vi "CRYUpdate Calibration Date.vi"(11 "Calibration In":T1 {"Calibration 2D"."Sens Curve"."Z data" items=["dB", "Lin"]; "Calibration 2D"."Sens Curve"."X data" items=["dB", "Lin"]; "Calibration 2D"."Sens Curve"."Y data" items=["dB", "Lin"]; "Calibration 2D"."Sens Curve"."Z dB ref" format="%.1f"; "Calibration 2D"."Sens Curve"."Z axis" items=["Log", "Lin"]; "Calibration 2D"."Sens Curve"."X dB ref" format="%.1f"; "Calibration 2D"."Sens Curve"."X axis" items=["Log", "Lin"]; "Calibration 2D"."Sens Curve"."Y axis" items=["Log", "Lin"]; "Calibration 2D"."Sens Curve"."Y dB ref" format="%.1f"; "Calibration 2D"."Sens Curve"."Curve"."z" format="%.2f"; "Calibration 2D"."Sens Curve"."Curve"."y" format="%.2f"; "Calibration 2D"."Sens Curve"."Curve"."x" format="%.2f"; "Calibration 2D"."EQ Curve"."Z data" items=["dB", "Lin"]; "Calibration 2D"."EQ Curve"."X data" items=["dB", "Lin"]; "Calibration 2D"."EQ Curve"."Y data" items=["dB", "Lin"]; "Calibration 2D"."EQ Curve"."Z dB ref" format="%.1f"; "Calibration 2D"."EQ Curve"."Z axis" items=["Log", "Lin"]; "Calibration 2D"."EQ Curve"."X dB ref" format="%.1f"; "Calibration 2D"."EQ Curve"."X axis" items=["Log", "Lin"]; "Calibration 2D"."EQ Curve"."Y axis" items=["Log", "Lin"]; "Calibration 2D"."EQ Curve"."Y dB ref" format="%.1f"; "Calibration 2D"."EQ Curve"."Curve"."z" format="%.2f"; "Calibration 2D"."EQ Curve"."Curve"."y" format="%.2f"; "Calibration 2D"."EQ Curve"."Curve"."x" format="%.2f"; "Calibration 2D"."Corr Curve"."Z data" items=["dB", "Lin"]; "Calibration 2D"."Corr Curve"."X data" items=["dB", "Lin"]; "Calibration 2D"."Corr Curve"."Y data" items=["dB", "Lin"]; "Calibration 2D"."Corr Curve"."Z dB ref" format="%.1f"; "Calibration 2D"."Corr Curve"."Z axis" items=["Log", "Lin"]; "Calibration 2D"."Corr Curve"."X dB ref" format="%.1f"; "Calibration 2D"."Corr Curve"."X axis" items=["Log", "Lin"]; "Calibration 2D"."Corr Curve"."Y axis" items=["Log", "Lin"]; "Calibration 2D"."Corr Curve"."Y dB ref" format="%.1f"; "Calibration 2D"."Corr Curve"."Curve"."z" format="%.2f"; "Calibration 2D"."Corr Curve"."Curve"."y" format="%.2f"; "Calibration 2D"."Corr Curve"."Curve"."x" format="%.2f"; "Calibration 2D"."Calibration"."EQ Step size" items=["R10", "R20", "R40", "R80", "User"]; "Calibration 2D"."Calibration"."Corr Step size" items=["R10", "R20", "R40", "R80", "User"]}) -> (3 "Calibration Out":T1 {"Calibration 2D"."Sens Curve"."Z data" items=["dB", "Lin"]; "Calibration 2D"."Sens Curve"."X data" items=["dB", "Lin"]; "Calibration 2D"."Sens Curve"."Y data" items=["dB", "Lin"]; "Calibration 2D"."Sens Curve"."Z dB ref" format="%.1f"; "Calibration 2D"."Sens Curve"."Z axis" items=["Log", "Lin"]; "Calibration 2D"."Sens Curve"."X dB ref" format="%.1f"; "Calibration 2D"."Sens Curve"."X axis" items=["Log", "Lin"]; "Calibration 2D"."Sens Curve"."Y axis" items=["Log", "Lin"]; "Calibration 2D"."Sens Curve"."Y dB ref" format="%.1f"; "Calibration 2D"."Sens Curve"."Curve"."z" format="%.2f"; "Calibration 2D"."Sens Curve"."Curve"."y" format="%.2f"; "Calibration 2D"."Sens Curve"."Curve"."x" format="%.2f"; "Calibration 2D"."EQ Curve"."Z data" items=["dB", "Lin"]; "Calibration 2D"."EQ Curve"."X data" items=["dB", "Lin"]; "Calibration 2D"."EQ Curve"."Y data" items=["dB", "Lin"]; "Calibration 2D"."EQ Curve"."Z dB ref" format="%.1f"; "Calibration 2D"."EQ Curve"."Z axis" items=["Log", "Lin"]; "Calibration 2D"."EQ Curve"."X dB ref" format="%.1f"; "Calibration 2D"."EQ Curve"."X axis" items=["Log", "Lin"]; "Calibration 2D"."EQ Curve"."Y axis" items=["Log", "Lin"]; "Calibration 2D"."EQ Curve"."Y dB ref" format="%.1f"; "Calibration 2D"."EQ Curve"."Curve"."z" format="%.2f"; "Calibration 2D"."EQ Curve"."Curve"."y" format="%.2f"; "Calibration 2D"."EQ Curve"."Curve"."x" format="%.2f"; "Calibration 2D"."Corr Curve"."Z data" items=["dB", "Lin"]; "Calibration 2D"."Corr Curve"."X data" items=["dB", "Lin"]; "Calibration 2D"."Corr Curve"."Y data" items=["dB", "Lin"]; "Calibration 2D"."Corr Curve"."Z dB ref" format="%.1f"; "Calibration 2D"."Corr Curve"."Z axis" items=["Log", "Lin"]; "Calibration 2D"."Corr Curve"."X dB ref" format="%.1f"; "Calibration 2D"."Corr Curve"."X axis" items=["Log", "Lin"]; "Calibration 2D"."Corr Curve"."Y axis" items=["Log", "Lin"]; "Calibration 2D"."Corr Curve"."Y dB ref" format="%.1f"; "Calibration 2D"."Corr Curve"."Curve"."z" format="%.2f"; "Calibration 2D"."Corr Curve"."Curve"."y" format="%.2f"; "Calibration 2D"."Corr Curve"."Curve"."x" format="%.2f"; "Calibration 2D"."Calibration"."EQ Step size" items=["R10", "R20", "R40", "R80", "User"]; "Calibration 2D"."Calibration"."Corr Step size" items=["R10", "R20", "R40", "R80", "User"]})   [LabVIEW 2013]
uses:
  Typedef Control/CRYCalibration All Cluster.ctl
  Typedef Control/CRYCalibration 2DCluster.ctl
  Typedef Control/CRYCalibration Cluster.ctl
  Typedef Control/CRYData Cluster.ctl
  CRYProject/CRYProject Editor Global.vi
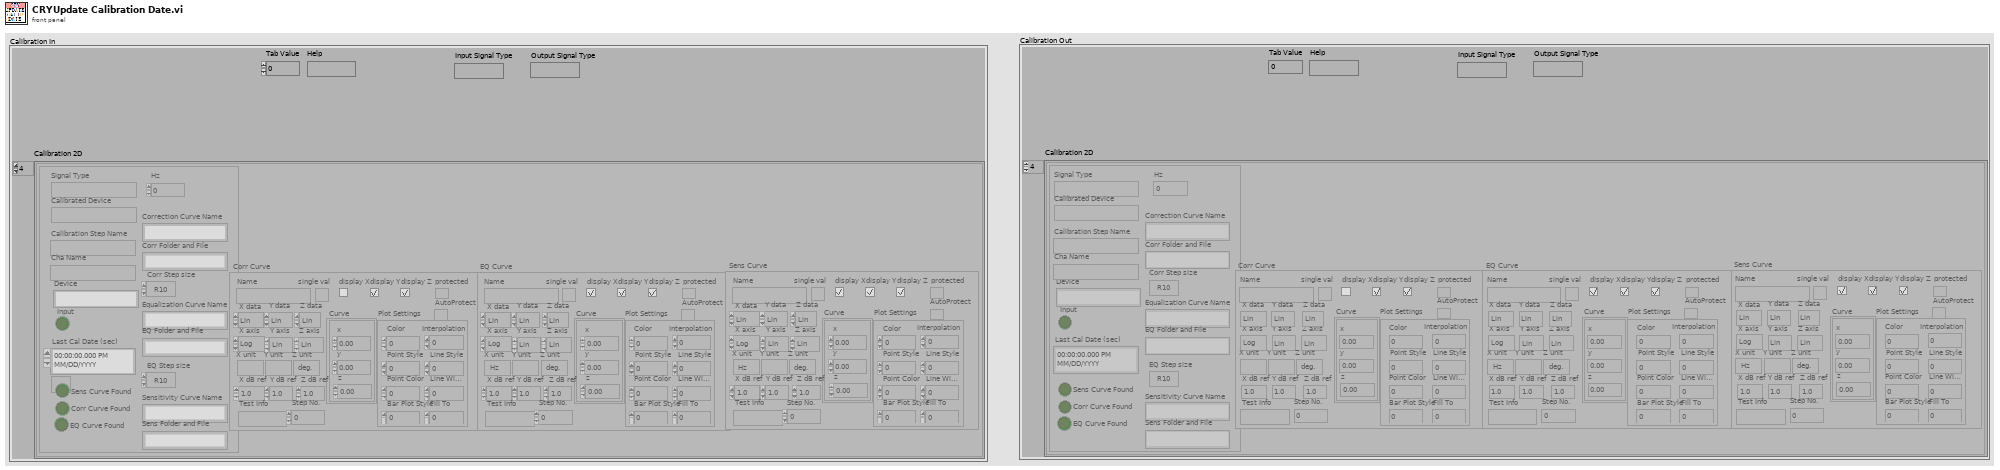
[diagram p1: front panel]
types:
  T1 = typedef "CRYCalibration All Cluster.ctl" = cluster{"Calibration 2D":T2[], "Help":string, "Tab Value":i32, "Input Signal Type":string, "Output Signal Type":string}
  T2 = typedef "CRYCalibration 2DCluster.ctl" = cluster{"Calibration":T3, "Corr Curve":T4, "EQ Curve":T4, "Sens Curve":T4}
  T3 = typedef "CRYCalibration Cluster.ctl" = cluster{"Calibration Step Name":string, "Device":string, "Correction Curve Name":string, "Equalization Curve Name":string, "Sensitivity Curve Name":string, "Corr Folder and File":string, "EQ Folder and File":string, "Sens Folder and File":string, "Corr Step size":u16, "EQ Step size":u16, "Input":bool, "Last Cal Date (sec)":timestamp, "Cha Name":string, "Corr Curve Found":bool, "EQ Curve Found":bool, "Sens Curve Found":bool, "Signal Type":string, "Calibrated Device":string, "Hz":u32}
  T4 = typedef "CRYData Cluster.ctl" = cluster{"Name":string, "Curve":cluster{"x":dbl, "y":dbl, "z":dbl}[], "X data":u16, "Y data":u16, "Z data":u16, "X axis":u16, "Y axis":u16, "Z axis":u16, "X unit":string, "Y unit":string, "Z unit":string, "X dB ref":dbl, "Y dB ref":dbl, "Z dB ref":dbl, "single val":bool, "protected":bool, "display X":bool, "display Y":bool, "display Z":bool, "Test Info":string, "Step No.":i32, "Plot Settings":cluster{"Color":u32, "Interpolation":u8, "Point Style":u8, "Line Style":u8, "Point Color":u32, "Line Width":u8, "Bar Plot Style":u8, "Fill To":i16}, "AutoProtect":bool}
  T5 = typedef "CRYStep.ctl" = cluster{"No.VI":i32, "Category":string, "StepName":string, "Seq setup flattened":string, "Comment":string, "Steps config.":bool[], "Jump config":i32[], "Start":dbl, "Increment":dbl, "Name":string, "Unit":string, "Y data":u16, "Y prefix":string, "Y dB ref":dbl, "Y unit":string, "Repeat State Array":cluster{"Start":dbl, "Increment":dbl, "Count":i32, "Num":i32}[]}
  T6 = cluster{"Calibration":cluster{"Calibration Step Name":bool, "Device":bool, "Correction Curve Name":bool, "Equalization Curve Name":bool, "Sensitivity Curve Name":bool, "Corr Folder and File":bool, "EQ Folder and File":bool, "Sens Folder and File":bool, "Corr Step size":bool, "EQ Step size":bool, "Input":bool, "Last Cal Date (sec)":bool, "Cha Name":bool, "Corr Curve Found":bool, "EQ Curve Found":bool, "Sens Curve Found":bool, "Signal Type":bool, "Calibrated Device":bool, "Hz":bool}, "Corr Curve":cluster{"Name":bool, "Curve":cluster{"x":bool, "y":bool, "z":bool}[], "X data":bool, "Y data":bool, "Z data":bool, "X axis":bool, "Y axis":bool, "Z axis":bool, "X unit":bool, "Y unit":bool, "Z unit":bool, "X dB ref":bool, "Y dB ref":bool, "Z dB ref":bool, "single val":bool, "protected":bool, "display X":bool, "display Y":bool, "display Z":bool, "Test Info":bool, "Step No.":bool, "Plot Settings":cluster{"Color":bool, "Interpolation":bool, "Point Style":bool, "Line Style":bool, "Point Color":bool, "Line Width":bool, "Bar Plot Style":bool, "Fill To":bool}, "AutoProtect":bool}, "EQ Curve":cluster{"Name":bool, "Curve":cluster{"x":bool, "y":bool, "z":bool}[], "X data":bool, "Y data":bool, "Z data":bool, "X axis":bool, "Y axis":bool, "Z axis":bool, "X unit":bool, "Y unit":bool, "Z unit":bool, "X dB ref":bool, "Y dB ref":bool, "Z dB ref":bool, "single val":bool, "protected":bool, "display X":bool, "display Y":bool, "display Z":bool, "Test Info":bool, "Step No.":bool, "Plot Settings":cluster{"Color":bool, "Interpolation":bool, "Point Style":bool, "Line Style":bool, "Point Color":bool, "Line Width":bool, "Bar Plot Style":bool, "Fill To":bool}, "AutoProtect":bool}, "Sens Curve":cluster{"Name":bool, "Curve":cluster{"x":bool, "y":bool, "z":bool}[], "X data":bool, "Y data":bool, "Z data":bool, "X axis":bool, "Y axis":bool, "Z axis":bool, "X unit":bool, "Y unit":bool, "Z unit":bool, "X dB ref":bool, "Y dB ref":bool, "Z dB ref":bool, "single val":bool, "protected":bool, "display X":bool, "display Y":bool, "display Z":bool, "Test Info":bool, "Step No.":bool, "Plot Settings":cluster{"Color":bool, "Interpolation":bool, "Point Style":bool, "Line Style":bool, "Point Color":bool, "Line Width":bool, "Bar Plot Style":bool, "Fill To":bool}, "AutoProtect":bool}}
  T7 = cluster{"Calibration Step Name":bool, "Device":bool, "Correction Curve Name":bool, "Equalization Curve Name":bool, "Sensitivity Curve Name":bool, "Corr Folder and File":bool, "EQ Folder and File":bool, "Sens Folder and File":bool, "Corr Step size":bool, "EQ Step size":bool, "Input":bool, "Last Cal Date (sec)":bool, "Cha Name":bool, "Corr Curve Found":bool, "EQ Curve Found":bool, "Sens Curve Found":bool, "Signal Type":bool, "Calibrated Device":bool, "Hz":bool}
  T8 = cluster{"Name":bool, "Curve":cluster{"x":bool, "y":bool, "z":bool}[], "X data":bool, "Y data":bool, "Z data":bool, "X axis":bool, "Y axis":bool, "Z axis":bool, "X unit":bool, "Y unit":bool, "Z unit":bool, "X dB ref":bool, "Y dB ref":bool, "Z dB ref":bool, "single val":bool, "protected":bool, "display X":bool, "display Y":bool, "display Z":bool, "Test Info":bool, "Step No.":bool, "Plot Settings":cluster{"Color":bool, "Interpolation":bool, "Point Style":bool, "Line Style":bool, "Point Color":bool, "Line Width":bool, "Bar Plot Style":bool, "Fill To":bool}, "AutoProtect":bool}
  T9 = cluster{"Color":bool, "Interpolation":bool, "Point Style":bool, "Line Style":bool, "Point Color":bool, "Line Width":bool, "Bar Plot Style":bool, "Fill To":bool}
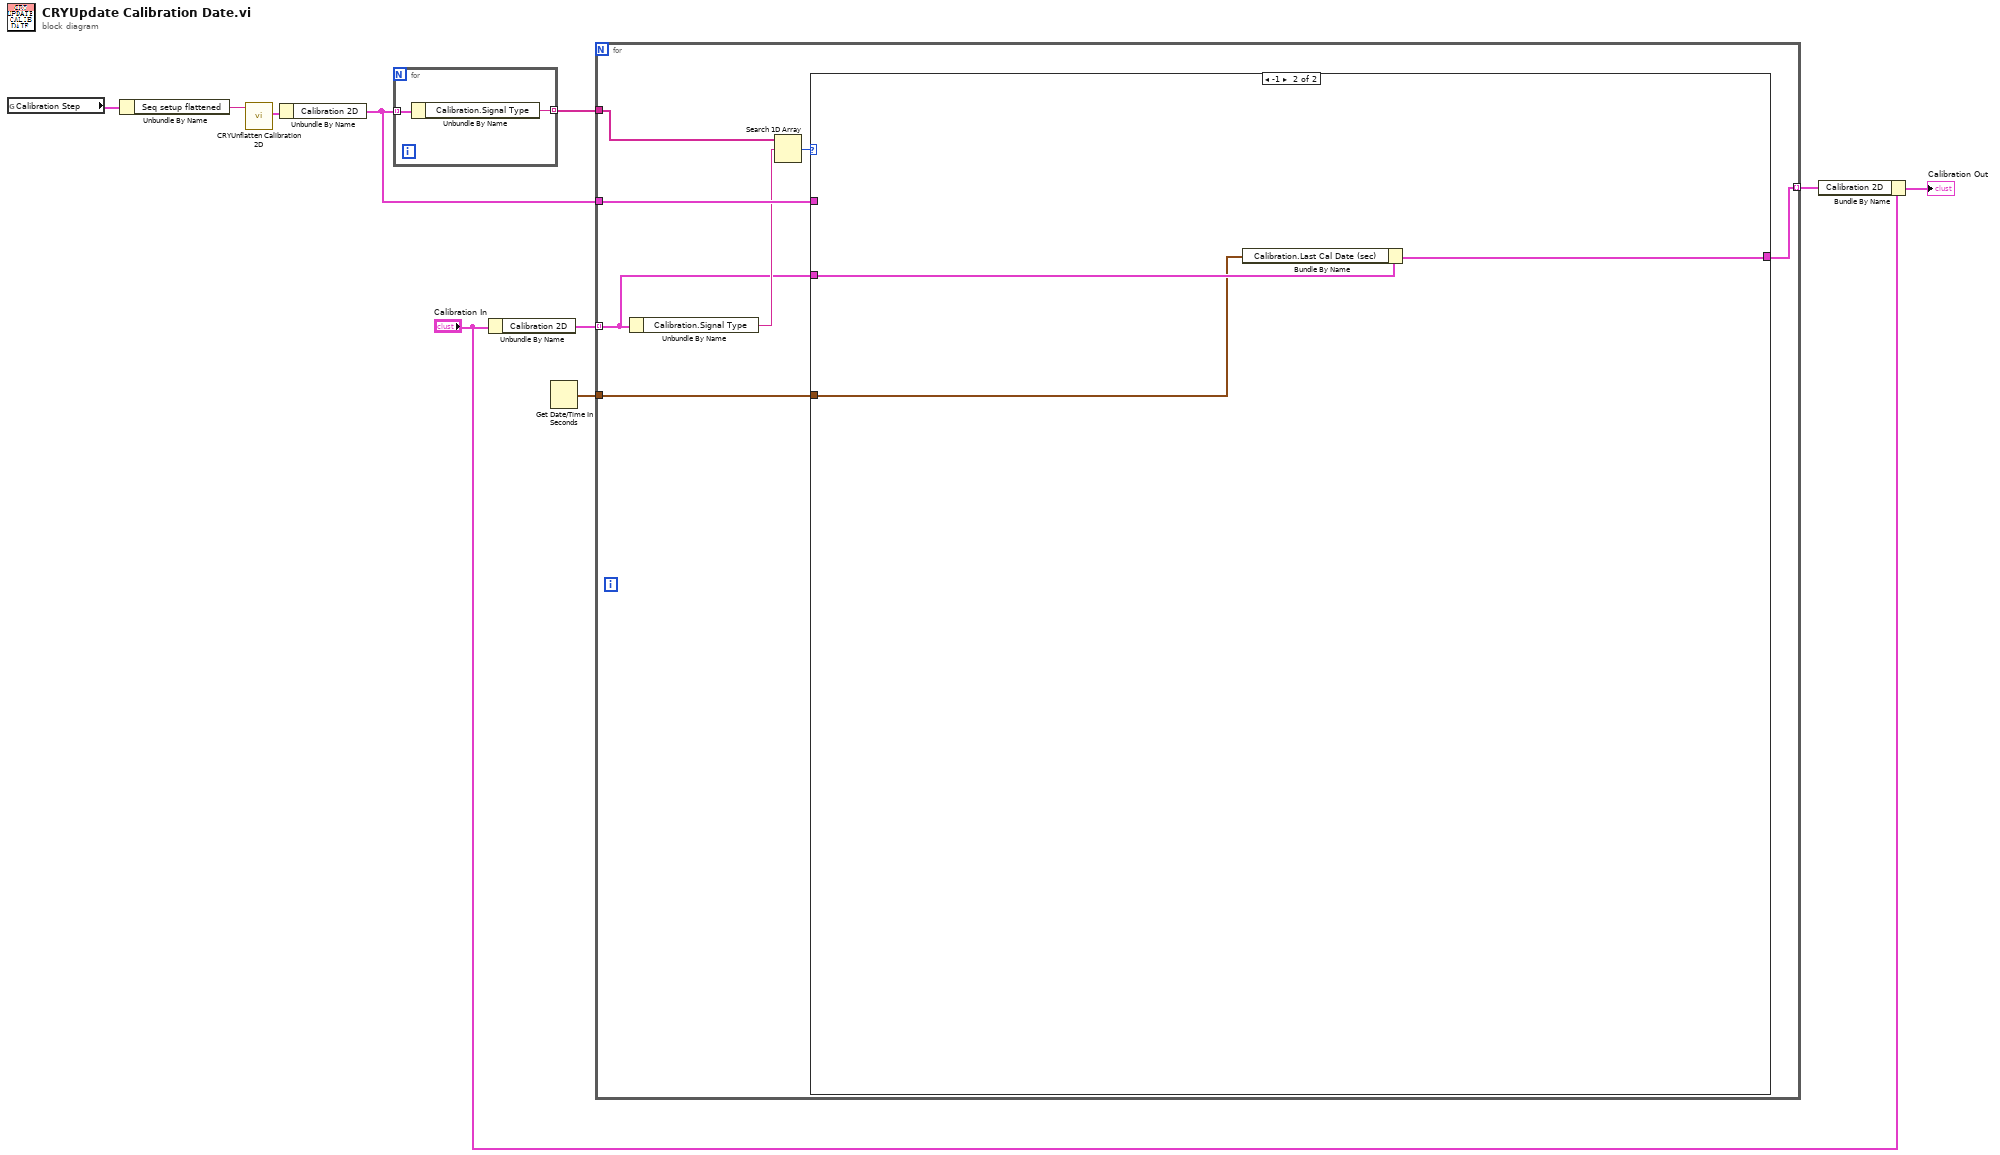
[diagram p0: block diagram]
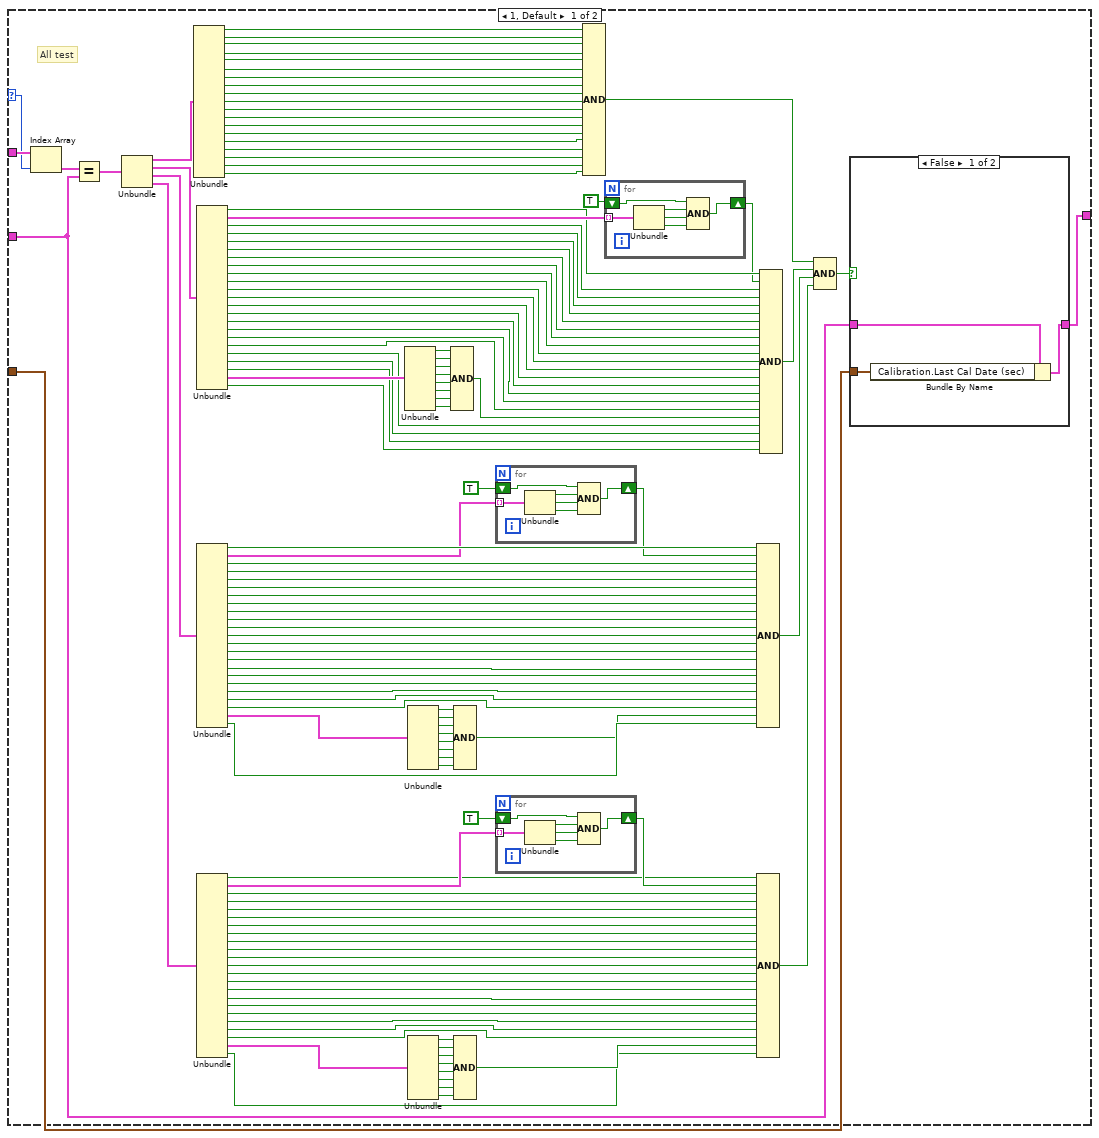
[diagram p2: hidden frame]
diagram:
  n1 = global read "CRYProject Editor Global.vi" "Calibration Step"() -> (w10:T5)
  n2 = Unbundle By Name(w10) -> ("Seq setup flattened"=w9:string)
  n3 = call "CRYUnflatten Calibration 2D.vi"("Flattened Calibration"=w9) -> ("Calibration Step Out"=w8:T1)  [unwired: 8 in, 2 out]
  n4 = Unbundle By Name(w8) -> ("Calibration 2D"=w6:T2[])
  n5 = for {
    tunnel: w6 -> [w12] mode=indexing
    tunnel: [w11] -> w5 mode=indexing
    n6 = Unbundle By Name(w12) -> ("Calibration.Signal Type"=w11:string)
  }
  n7 = Unbundle By Name("Calibration In") -> ("Calibration 2D"=w7:T2[])
  n8 = Get Date/Time In Seconds() -> (seconds since 1Jan1904=w1:timestamp)
  n9 = for {
    tunnel: w7 -> [w14] mode=indexing
    tunnel: w6 -> [w19]
    tunnel: w5 -> [w18]
    tunnel: [w13] -> w4 mode=indexing
    tunnel: w1 -> [w15]
    n10 = Unbundle By Name(w14) -> ("Calibration.Signal Type"=w17:string)
    n11 = Search 1D Array(1D array=w18, element=w17) -> (index of element=w16:i32)  [unwired: 1 in]
    n12 = case shown="-1" w16 {
      selector: w16 -> [w155 _]
      tunnel: w19 -> [w156 _]
      tunnel: w14 -> [w152 w181]
      tunnel: w15 -> [w154 w180]
      tunnel: [w151 w179] -> w13
      frame 1, Default {
        # "All test"
        n13 = Index Array(array=w156, index=w155) -> (element=w153:T2)
        n14 = Equal?(x=w153, y=w152) -> (x = y?=w150:T6)
        n15 = Unbundle(w150) -> ("Calibration"=w149:T7, "Corr Curve"=w148:T8, "EQ Curve"=w147:T8, "Sens Curve"=w22:T8)
        n16 = Unbundle(w149) -> ("Calibration Step Name"=w145:bool, "Device"=w144:bool, "Correction Curve Name"=w143:bool, "Equalization Curve Name"=w142:bool, "Sensitivity Curve Name"=w141:bool, "Corr Folder and File"=w140:bool, "EQ Folder and File"=w139:bool, "Sens Folder and File"=w138:bool, "Corr Step size"=w137:bool, "EQ Step size"=w136:bool, "Input"=w135:bool, "Last Cal Date (sec)"=w134:bool, "Cha Name"=w133:bool, "Corr Curve Found"=w132:bool, "EQ Curve Found"=w131:bool, "Sens Curve Found"=w130:bool, "Signal Type"=w129:bool, "Calibrated Device"=w128:bool, "Hz"=w127:bool)
        n17 = Unbundle(w148) -> ("Name"=w124:bool, "Curve"=w146:cluster{"x":bool, "y":bool, "z":bool}[], "X data"=w122:bool, "Y data"=w121:bool, "Z data"=w120:bool, "X axis"=w119:bool, "Y axis"=w118:bool, "Z axis"=w117:bool, "X unit"=w108:bool, "Y unit"=w107:bool, "Z unit"=w106:bool, "X dB ref"=w105:bool, "Y dB ref"=w104:bool, "Z dB ref"=w103:bool, "single val"=w102:bool, "protected"=w101:bool, "display X"=w100:bool, "display Y"=w99:bool, "display Z"=w95:bool, "Test Info"=w98:bool, "Step No."=w97:bool, "Plot Settings"=w126:T9, "AutoProtect"=w96:bool)
        n18 = Unbundle(w147) -> ("Name"=w82:bool, "Curve"=w81:cluster{"x":bool, "y":bool, "z":bool}[], "X data"=w79:bool, "Y data"=w66:bool, "Z data"=w65:bool, "X axis"=w64:bool, "Y axis"=w63:bool, "Z axis"=w62:bool, "X unit"=w61:bool, "Y unit"=w60:bool, "Z unit"=w59:bool, "X dB ref"=w58:bool, "Y dB ref"=w68:bool, "Z dB ref"=w69:bool, "single val"=w70:bool, "protected"=w71:bool, "display X"=w72:bool, "display Y"=w73:bool, "display Z"=w74:bool, "Test Info"=w75:bool, "Step No."=w76:bool, "Plot Settings"=w83:T9, "AutoProtect"=w78:bool)
        n19 = Unbundle(w22) -> ("Name"=w32:bool, "Curve"=w33:cluster{"x":bool, "y":bool, "z":bool}[], "X data"=w35:bool, "Y data"=w48:bool, "Z data"=w49:bool, "X axis"=w50:bool, "Y axis"=w51:bool, "Z axis"=w52:bool, "X unit"=w53:bool, "Y unit"=w54:bool, "Z unit"=w55:bool, "X dB ref"=w56:bool, "Y dB ref"=w46:bool, "Z dB ref"=w45:bool, "single val"=w44:bool, "protected"=w43:bool, "display X"=w42:bool, "display Y"=w41:bool, "display Z"=w40:bool, "Test Info"=w39:bool, "Step No."=w38:bool, "Plot Settings"=w31:T9, "AutoProtect"=w36:bool)
        n20 = Unbundle(w126) -> ("Color"=w116:bool, "Interpolation"=w115:bool, "Point Style"=w114:bool, "Line Style"=w113:bool, "Point Color"=w112:bool, "Line Width"=w111:bool, "Bar Plot Style"=w110:bool, "Fill To"=w109:bool)
        n21 = Unbundle(w83) -> ("Color"=w84:bool, "Interpolation"=w85:bool, "Point Style"=w86:bool, "Line Style"=w87:bool, "Point Color"=w88:bool, "Line Width"=w89:bool, "Bar Plot Style"=w90:bool, "Fill To"=w91:bool)
        n22 = Unbundle(w31) -> ("Color"=w30:bool, "Interpolation"=w29:bool, "Point Style"=w28:bool, "Line Style"=w27:bool, "Point Color"=w26:bool, "Line Width"=w25:bool, "Bar Plot Style"=w24:bool, "Fill To"=w23:bool)
        n23 = Compound Arithmetic op=AND(w116, w115, w114, w113, w112, w111, w110, w109) -> (w94:bool)
        n24 = Compound Arithmetic op=AND(w84, w85, w86, w87, w88, w89, w90, w91) -> (w77:bool)
        n25 = Compound Arithmetic op=AND(w30, w29, w28, w27, w26, w25, w24, w23) -> (w37:bool)
        n26 = for {
          tunnel: w81 -> [w168] mode=indexing
          shift-right: [w163] -> w80
          shift-left: TRUE ("result") -> [w164]
          n27 = Unbundle(w168) -> ("x"=w167:bool, "y"=w166:bool, "z"=w165:bool)
          n28 = Compound Arithmetic op=AND(w164, w167, w166, w165) -> (w163:bool)
        }
        n29 = for {
          tunnel: w33 -> [w162] mode=indexing
          shift-right: [w157] -> w34
          shift-left: TRUE ("result") -> [w158]
          n30 = Unbundle(w162) -> ("x"=w161:bool, "y"=w160:bool, "z"=w159:bool)
          n31 = Compound Arithmetic op=AND(w158, w161, w160, w159) -> (w157:bool)
        }
        n32 = Compound Arithmetic op=AND(w145, w144, w143, w142, w141, w140, w139, w138, w137, w136, w135, w134, w133, w132, w131, w130, w129, w128, w127) -> (w93:bool)
        n33 = for {
          tunnel: w146 -> [w174] mode=indexing
          shift-right: [w169] -> w123
          shift-left: TRUE ("result") -> [w170]
          n34 = Unbundle(w174) -> ("x"=w173:bool, "y"=w172:bool, "z"=w171:bool)
          n35 = Compound Arithmetic op=AND(w170, w173, w172, w171) -> (w169:bool)
        }
        n36 = Compound Arithmetic op=AND(w82, w80, w79, w66, w65, w64, w63, w62, w61, w60, w59, w58, w68, w69, w70, w71, w72, w73, w74, w75, w76, w77, w78) -> (w57:bool)
        n37 = Compound Arithmetic op=AND(w32, w34, w35, w48, w49, w50, w51, w52, w53, w54, w55, w56, w46, w45, w44, w43, w42, w41, w40, w39, w38, w37, w36) -> (w21:bool)
        n38 = Compound Arithmetic op=AND(w124, w123, w122, w121, w120, w119, w118, w117, w108, w107, w106, w105, w104, w103, w102, w101, w100, w99, w94, w95, w98, w97, w96) -> (w92:bool)
        n39 = Compound Arithmetic op=AND(w93, w92, w57, w21) -> (w20:bool)
        n40 = case shown="False" w20 {
          tunnel: w152 -> [w177 w178]
          tunnel: [w176 w178] -> w151
          tunnel: w154 -> [w175 _]
          frame False {
            n41 = Bundle By Name(cluster=w177, "Calibration.Last Cal Date (sec)"=w175) -> (w176:T2)
          }
          frame True {
          }
        }
      }
      frame -1 {
        n42 = Bundle By Name(cluster=w181, "Calibration.Last Cal Date (sec)"=w180) -> (w179:T2)
      }
    }
  }
  n43 = Bundle By Name(cluster="Calibration In", "Calibration 2D"=w4) -> (→"Calibration Out":T1)
